vi "Camera Floc Interface.vi"(4 "State":i16, 5 "Time":dbl format="%.2f", 6 "Sensor Values":dbl[](array[numeric]), 7 "Set Points":dbl[](array[numeric])=[1.0]) -> (0 "required data":T3, 3 "output value":dbl)   [LabVIEW 2012]
uses:
  <vilib>/userdefined/High Color/IMAQdx.ctl
  Camera source code/Interface Inputs.ctl
  Camera SubVIs.lvlib
  <vilib>/vision/driver/NI_Vision_Acquisition_Software.lvlib
panel:
  out "Image Save Rate (s)":dbl
  out "Interface inputs":T1={"Elevation of top of Field of View (cm)"=10.0, "Field of View Height (cm)"=-0.1, "Smooth Length (cm)"=5.0, "Min derivative magnitude"=5.0, "Color Plane"=enum."Green"} {"Smooth Length (cm)" min=0.01 max=1000.0 step=0.1; "Field of View Height (cm)" min=0.1 max=1000.0 step=0.1}
  out "error out":errorcluster
  out "Session Out":T2
  # "Enter the correct information for this control code in the required data structure below. Then make the current value default by right clicking on the border of the data structure. Select \"data operations\" and then select \"make current value default\". These values will be displayed by process controller."
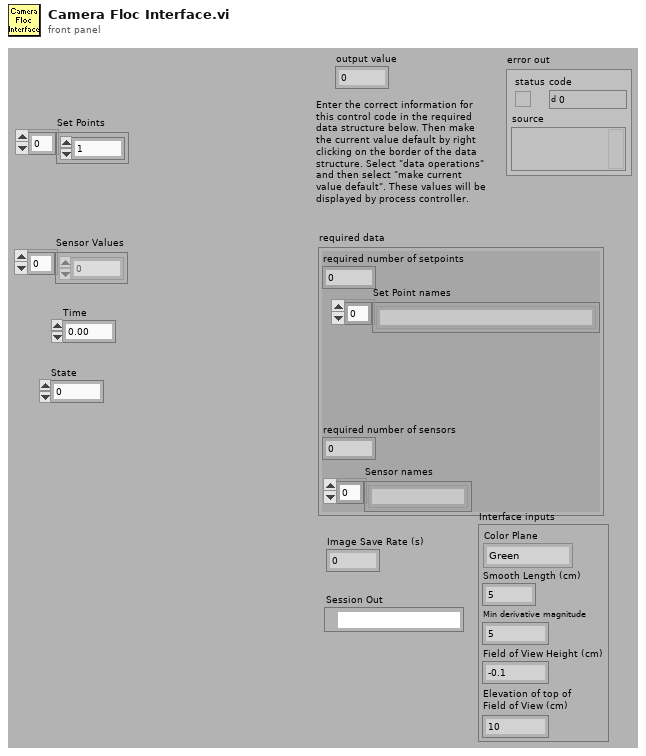
[diagram p1: front panel]
types:
  T1 = typedef "Camera SubVIs.lvlib/Interface Inputs.ctl" = cluster{"Elevation of top of Field of View (cm)":dbl, "Field of View Height (cm)":dbl, "Smooth Length (cm)":dbl, "Min derivative magnitude":dbl, "Color Plane":enum16{"Red", "Green", "Blue", "Combined"}}
  T2 = typedef "IMAQdx.ctl" = refnum<k21>
  T3 = cluster{"Set Point names":string[], "required number of setpoints":u8, "required number of sensors":u8, "Sensor names":string[]}
  T4 = typedef "Image Type" = u32
  T5 = cluster{"Global Rectangle":i32[], "Contours":cluster{"Contour Type":u32, "ROI Type":u32, "Points":i32[]}[]}
  T6 = typedef "Camera SubVIs.lvlib/Image File Type.ctl" = enum16{"BMP", "JPEG", "JPEG 2000", "PNG", "PNG with Vision Info", "TIFF"}
  T7 = typedef "Camera SubVIs.lvlib/Rotate.ctl" = enum16{"None", "CW", "CCW"}
  T8 = typedef "IMAQ Image.ctl" = refnum<image>
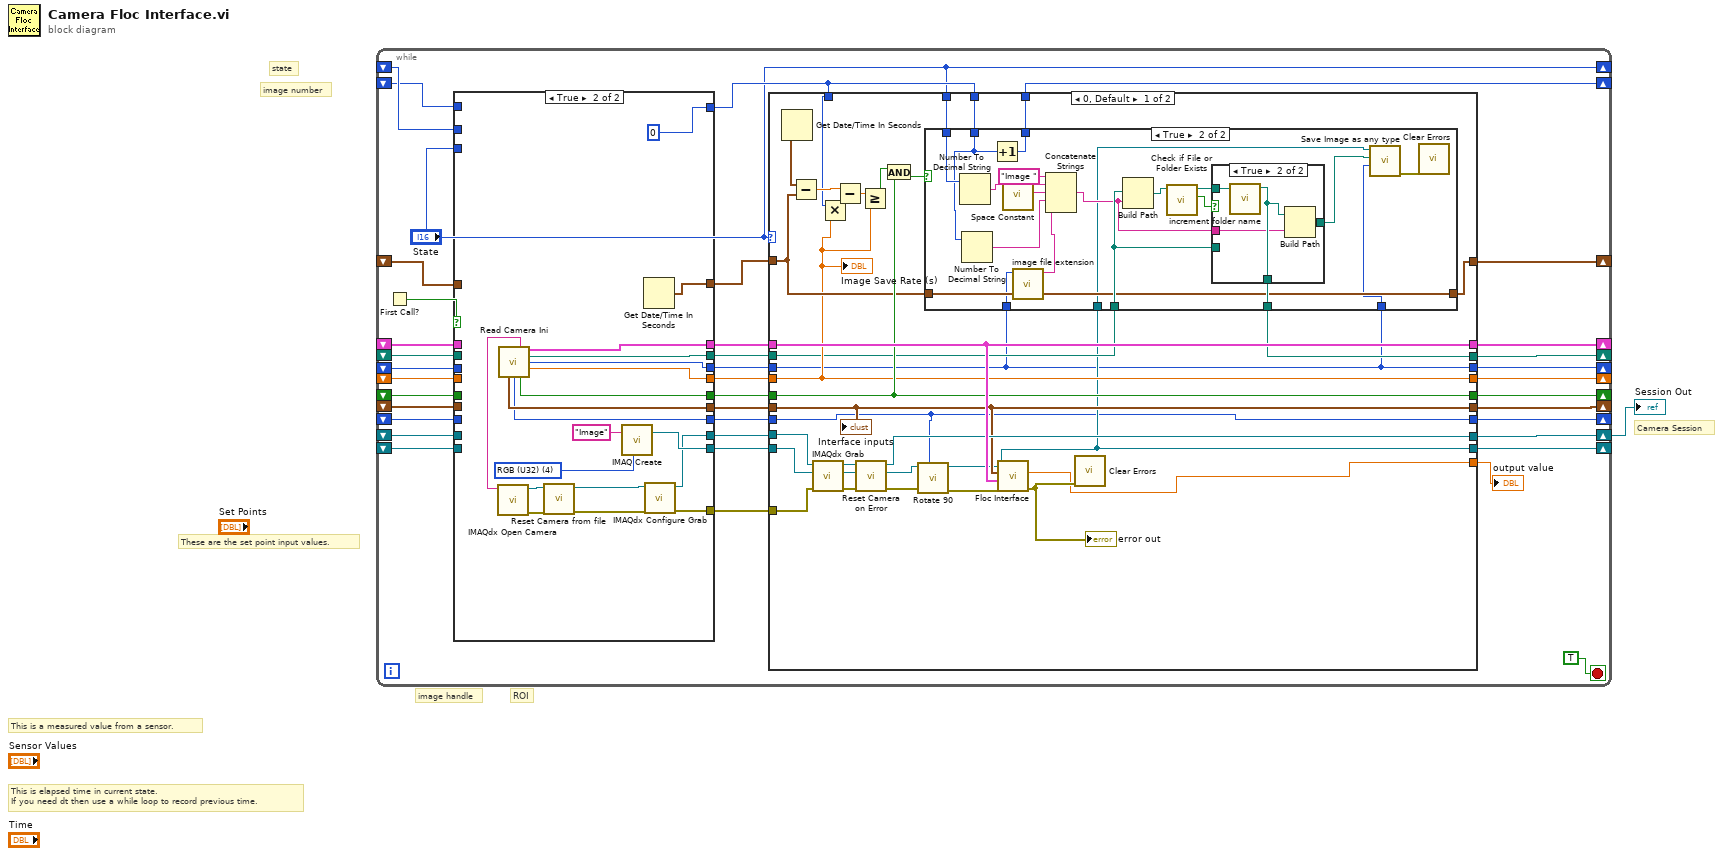
[diagram p0: block diagram]
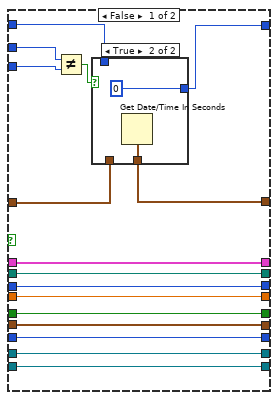
[diagram p2: hidden frame]
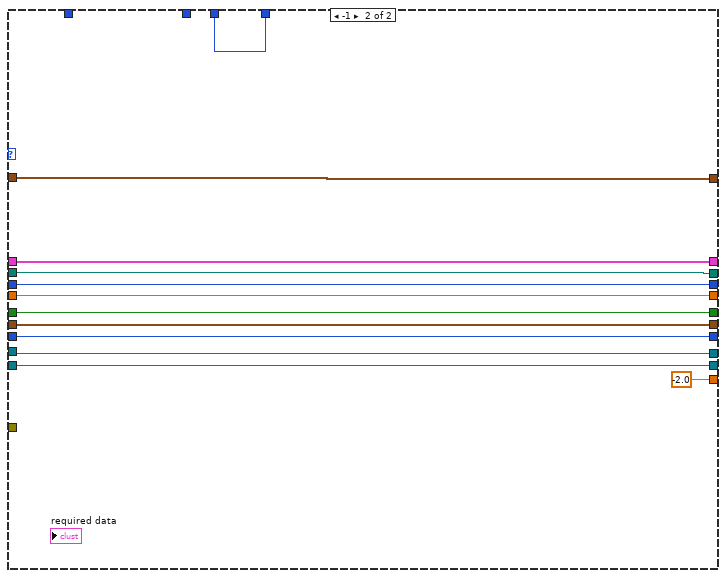
[diagram p6: hidden frame]
diagram:
  # "These are the set point input values."
  # "state"
  # "image number"
  # "ROI"
  # "image handle"
  # "Camera Session"
  # "This is a measured value from a sensor."
  # "This is elapsed time in current state.\nIf you need dt then use a while loop to record previous time."
  n1 = while {
    shift-right: [w38] -> w1
    shift-left: _ -> [w32]
    shift-right: [w19] -> _
    shift-left: _ -> [w36]
    shift-right: [w34] -> _
    shift-left: _ -> [w33]
    shift-right: [w30] -> _
    shift-left: _ -> [w24]
    shift-right: [w29] -> _
    shift-left: _ -> [w23]
    shift-right: [w28] -> _
    shift-left: _ -> [w22]
    shift-right: [w21] -> _
    shift-left: _ -> [w10]
    shift-right: ["State"] -> _
    shift-left: _ -> [w12]
    shift-right: [w20] -> _
    shift-left: _ -> [w9]
    shift-right: [w18] -> _
    shift-left: _ -> [w16]
    shift-right: [w6] -> _
    shift-left: _ -> [w5]
    shift-right: [w3] -> _
    shift-left: _ -> [w2]
    stop <- TRUE stop-if-true
    n2 = First Call?() -> (First Call?: T/F=w15:bool)
    n3 = case shown="True" w15 {
      tunnel: [w56 w77] -> w37
      tunnel: w36 -> [w56 _]
      tunnel: [w55 w76] -> w35
      tunnel: w33 -> [w55 _]
      tunnel: w32 -> [w54 _]
      tunnel: [w54 w68] -> w31
      tunnel: [w53 w75] -> w27
      tunnel: [w52 w74] -> w26
      tunnel: [w51 w73] -> w25
      tunnel: w24 -> [w53 _]
      tunnel: w23 -> [w52 _]
      tunnel: w22 -> [w51 _]
      tunnel: [w50 w72] -> w17
      tunnel: w16 -> [w50 _]
      tunnel: [w47 0] -> w14
      tunnel: [w46 w66] -> w13
      tunnel: w12 -> [w49 _]
      tunnel: "State" -> [w48 _]
      tunnel: w10 -> [w45 _]
      tunnel: w9 -> [w44 _]
      tunnel: [_ w63] -> w8
      tunnel: [w42 w62] -> w7
      tunnel: w5 -> [w42 _]
      tunnel: [w41 w61] -> w4
      tunnel: w2 -> [w41 _]
      frame False {
        n4 = Not Equal?(x=w49, y=w48) -> (x != y?=w43:bool)
        n5 = case shown="True" w43 {
          tunnel: [w58 0] -> w47
          tunnel: w44 -> [w58 _]
          tunnel: [w57 w59] -> w46
          tunnel: w45 -> [w57 _]
          frame False {
          }
          frame True {
            n6 = Get Date/Time In Seconds() -> (seconds since 1Jan1904=w59:timestamp)
          }
        }
      }
      frame True {
        w79 = T4 4 items=["Grayscale (U8)", "Grayscale (I16)", "Grayscale (SGL)", "Complex (CSG)", "RGB (U32)", "HSL (U32)", "RGB (U64)", "Grayscale (U16)"] ("Image Type")
        n7 = call "Read Camera Ini.vi"() -> ("CameraName"=w71:string, "ROI"=w76:T5, "Image folder"=w75:path, "File Type"=w62:T6, "Image Save Rate (s)"=w74:dbl, "Interface inputs"=w72:T1, "Rotate"=w61:T7, "Record images"=w73:bool)  [unwired: 7 in, 1 out]
        n8 = call <vilib>:"IMAQdx Open Camera.vi"("Session In"=w71) -> ("error out"=w65:errorcluster, "Session Out"=w70:T2)  [unwired: 9 in]
        n9 = call "Reset Camera from file.vi"("error in"=w65, "Refnum in"=w70) -> ("error out"=w64:errorcluster, "Refnum out"=w69:T2)  [unwired: 8 in]
        n10 = call "IMAQ Create"("Image Name"="Image", "Image Type"=w79) -> ("New Image"=w77:T8)  [unwired: 2 in, 2 out]
        n11 = Get Date/Time In Seconds() -> (seconds since 1Jan1904=w66:timestamp)
        n12 = call <vilib>:"IMAQdx Configure Grab.vi"("error in"=w64, "Session In"=w69) -> ("error out"=w63:errorcluster, "Session Out"=w68:T2)  [unwired: 8 in]
      }
    }
    n13 = case shown="0, Default" "State" {
      tunnel: [w89 -2.0 ("fraction on")] -> w40
      tunnel: [w107 w144] -> w38
      tunnel: w31 -> [w112 w144]
      tunnel: w37 -> [w91 w145]
      tunnel: [w82 w145] -> w19
      tunnel: w35 -> [w111 w152]
      tunnel: [w111 w152] -> w34
      tunnel: [w92 w151] -> w30
      tunnel: [w95 w150] -> w29
      tunnel: [w106 w149] -> w28
      tunnel: w27 -> [w93 w151]
      tunnel: w26 -> [w95 w150]
      tunnel: w25 -> [w106 w149]
      tunnel: w13 -> [w100 w148]
      tunnel: [w105 w148] -> w21
      tunnel: w14 -> [w103 w147]
      tunnel: [w102 w147] -> w20
      tunnel: "State" -> [w101 _]
      tunnel: w14 -> [w94 _]
      tunnel: [w88 w146] -> w18
      tunnel: w17 -> [w88 w146]
      tunnel: w8 -> [w86 _]
      tunnel: w7 -> [w80 w143]
      tunnel: [w80 w143] -> w6
      tunnel: [w81 w142] -> w3
      tunnel: w4 -> [w81 w142]
      frame 0, Default {
        n14 = Get Date/Time In Seconds() -> (seconds since 1Jan1904=w87:timestamp)
        n15 = Subtract(x=w87, y=w100) -> (x-y=w99:dbl)
        n16 = call <vilib>:"IMAQdx Grab.vi"("error in"=w86, "Image In"=w91, "Session In"=w112) -> ("error out"=w109:errorcluster, "Image Out"=w90:T8, "Session Out"=w108:T2)  [unwired: 5 in, 1 out]
        n17 = Multiply(x=w94, y=w95) -> (x*y=w98:dbl)
        n18 = Subtract(x=w99, y=w98) -> (x-y=w96:dbl)
        n19 = call "Reset Camera on Error.vi"("error in"=w109, "Image in"=w90, "Session in"=w108) -> ("error out"=w85:errorcluster, "Image out"=w83:T8, "Session out"=w107:T2)  [unwired: 6 in]
        n20 = Greater Or Equal?(x=w96, y=w95) -> (x >= y?=w97:bool)
        n21 = And(x=w97, y=w106) -> (x .and. y?=w104:bool)
        n22 = call "Rotate 90.vi"("Rotate"=w81, "error in (no error)"=w85, "Image Src"=w83) -> ("error out"=w84:errorcluster, "Image Dst Out"=w82:T8)  [unwired: 7 in]
        n23 = case shown="True" w104 {
          tunnel: w100 -> [w115 w122]
          tunnel: [w115 w122] -> w105
          tunnel: w82 -> [_ w121]
          tunnel: w93 -> [w113 w128]
          tunnel: w103 -> [w114 w130]
          tunnel: [w114 w135] -> w102
          tunnel: w101 -> [_ w133]
          tunnel: [w113 w125] -> w92
          tunnel: w80 -> [_ w118]
          tunnel: w80 -> [_ w117]
          frame False {
          }
          frame True {
            n24 = Number To Decimal String(number=w133) -> (decimal integer string=w132:string)  [unwired: 1 in]
            n25 = Number To Decimal String(number=w130) -> (decimal integer string=w129:string)  [unwired: 1 in]
            n26 = Increment(x=w130) -> (x+1=w135:i32)
            n27 = call <vilib>:"Space Constant.vi"() -> ("String"=w131:string)
            n28 = call "image file extension.vi"("File Type"=w117) -> ("Extension"=w116:string)  [unwired: 10 in]
            n29 = Concatenate Strings("Image " ("string"), w132, w131, w129, w116) -> (w124:string)
            n30 = Build Path(base path=w128, name or relative path=w124) -> (appended path=w123:path)
            n31 = call <vilib>:"Check if File or Folder Exists.vi"("path"=w123) -> ("file or folder exists?"=w127:bool, "dup path"=w126:path)  [unwired: 8 in, 1 out]
            n32 = case shown="True" w127 {
              tunnel: w128 -> [w137 _]
              tunnel: w126 -> [w136 w141]
              tunnel: [w137 w140] -> w125
              tunnel: w124 -> [_ w139]
              tunnel: [w136 w138] -> w120
              frame False {
              }
              frame True {
                n33 = call "increment folder name.vi"("Image folder"=w141) -> ("appended path"=w140:path)  [unwired: 10 in]
                n34 = Build Path(base path=w140, name or relative path=w139) -> (appended path=w138:path)
              }
            }
            n35 = call "Save Image as any type.vi"("File Type"=w118, "File Path"=w120, "Image"=w121) -> ("error out"=w119:errorcluster)  [unwired: 7 in, 1 out]
            n36 = call <vilib>:"Clear Errors.vi"("error in (no error)"=w119) -> ()  [unwired: 6 in, 1 out]
          }
        }
        n37 = call "Floc Interface.vi"("error in"=w84, "ROI"=w111, "Interface inputs"=w88, "Image"=w82) -> ("error out"=w110:errorcluster, "Interface elevation"=w89:dbl)  [unwired: 4 in, 2 out]
        "error out" <- w110
        n38 = call <vilib>:"Clear Errors.vi"("error in (no error)"=w110) -> ()  [unwired: 6 in, 1 out]
        "Interface inputs" <- w88
        "Image Save Rate (s)" <- w95
      }
      frame -1 {
      }
    }
    "output value" <- w40
  }
  "Session Out" <- w1
